vi "Odd_Integar_Search.vi"() -> ()   [LabVIEW 2022 SP3]
panel:
  out "Divisible by 3":dbl
  out "Greater than 4000":dbl
  # "Odd_Integar_Search:\nThis program will find the smallest odd integars\nwhich are divisible by 3 and greater than 4000\nwhen cubed."
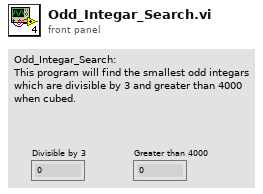
[diagram p1: front panel]
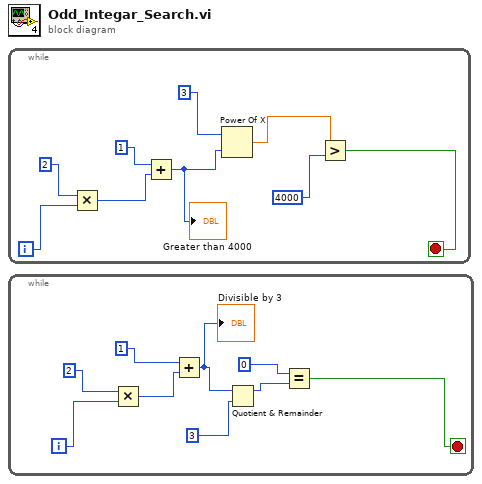
[diagram p0: block diagram]
diagram:
  n1 = while {
    i -> [w8]
    stop <- w2 stop-if-true
    n2 = Multiply(x=2, y=w8) -> (x*y=w7:i32)
    n3 = Add(x=1, y=w7) -> (x+y=w1:i32)
    "Greater than 4000" <- w1
    n4 = Power Of X(1:w1, 2:3) -> (0:w5:dbl)
    n5 = Greater?(x=w5, y=4000) -> (0:w2:bool)
  }
  n6 = while {
    i -> [w17]
    stop <- w11 stop-if-true
    n7 = Multiply(x=2, y=w17) -> (x*y=w15:i32)
    n8 = Add(x=1, y=w15) -> (x+y=w10:i32)
    "Divisible by 3" <- w10
    n9 = Quotient & Remainder(x=w10, y=3) -> (x-y*floor(x/y)=w13:i32)  [unwired: 1 out]
    n10 = Equal?(x=0, y=w13) -> (x = y?=w11:bool)
  }
